vi "GetFlattenedString.vi"(8 "error in":errorcluster, 11 "DateTime in":refnum<class "DateTime.lvclass">) -> (0 "error out":errorcluster, 2 "FlattenedString":string, 3 "DateTime out":refnum<class "DateTime.lvclass">)   [LabVIEW 2021, in "ProligentXMLGenerator.lvlib" / "DateTime.lvclass"]
uses:
  DateTime.lvclass
  DateTime.lvclass/DateTime.ctl
  ProligentXMLGenerator.lvlib
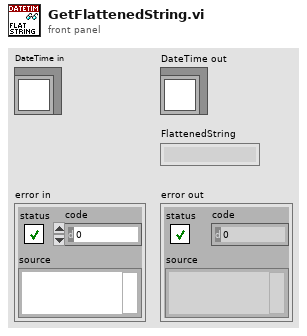
[diagram p1: front panel]
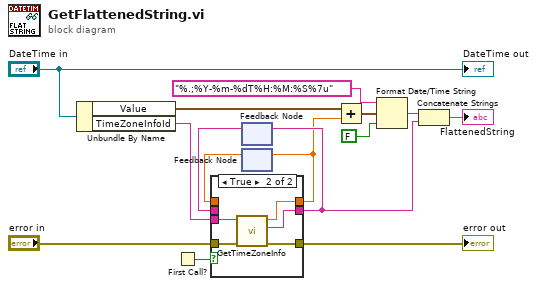
[diagram p0: block diagram]
diagram:
  n1 = Unbundle By Name("DateTime in") -> ("Value"=w4:timestamp, "TimeZoneInfoId"=w12:string)
  n2 = First Call?() -> (First Call?: T/F=w11:bool)
  n3 = feedback #1() -> (w9:string)  [unwired: 1 in]
  n4 = feedback #2() -> (w10:dbl)  [unwired: 1 in]
  n5 = case shown="True" w11 {
    tunnel: "error in" -> [w16 w23]
    tunnel: [w16 w22] -> w13
    tunnel: w12 -> [_ w21]
    tunnel: [w18 w20] -> w2
    tunnel: [w17 w19] -> w3
    tunnel: w10 -> [w18 _]
    tunnel: w9 -> [w17 _]
    frame False {
    }
    frame True {
      n6 = call "GetTimeZoneInfo.vi"("error in"=w23, "TimeZoneInfoId"=w21) -> ("error out"=w22:errorcluster, "OffsetSuffix"=w19:string, "Offset"=w20:dbl)  [unwired: 7 in]
    }
  }
  "error out" <- w13
  n7 = feedback-in #1(w3) -> ()
  n8 = feedback-in #2(w2) -> ()
  n9 = Add(x=w4, y=w2) -> (x+y=w7:timestamp)
  n10 = Format Date/Time String(time format string (%c)="%.;%Y-%m-%dT%H:%M:%S%7u", seconds (now)=w7, UTC format=FALSE) -> (date/time string=w5:string)
  n11 = Concatenate Strings(w5, w3) -> (→"FlattenedString":string)
  "DateTime out" <- "DateTime in"
